vi "Process Message.vi"(8 "error in (no error)":errorcluster, 11 "Message Transport in":refnum<class "Message Transport.lvclass">) -> (0 "error out":errorcluster, 2 "Action":refnum<class "Action.lvclass">, 3 "Message Transport out":refnum<class "Message Transport.lvclass">)   [LabVIEW 2018, in "Message Transport.lvclass"]
uses:
  Message Transport.lvclass
  Action_class/Action.lvclass
  Message Transport.lvclass/Message Transport.ctl
  Message_class/Message.lvclass/Message.ctl
  Communication_class/Get Message Queue.vi
  Message_class/Get Action.vi
  Message_class/Message.lvclass
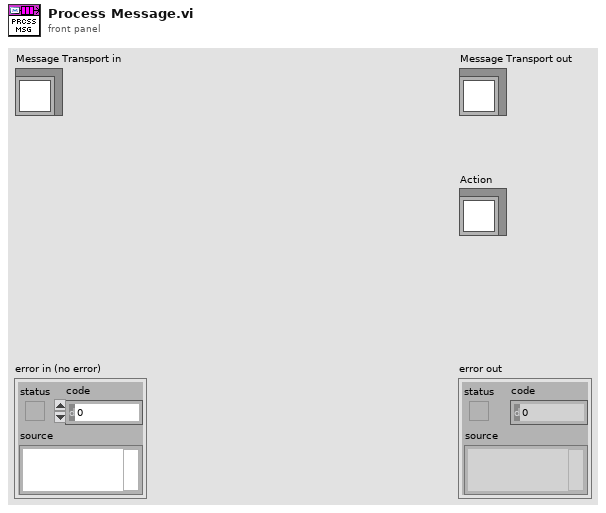
[diagram p1: front panel]
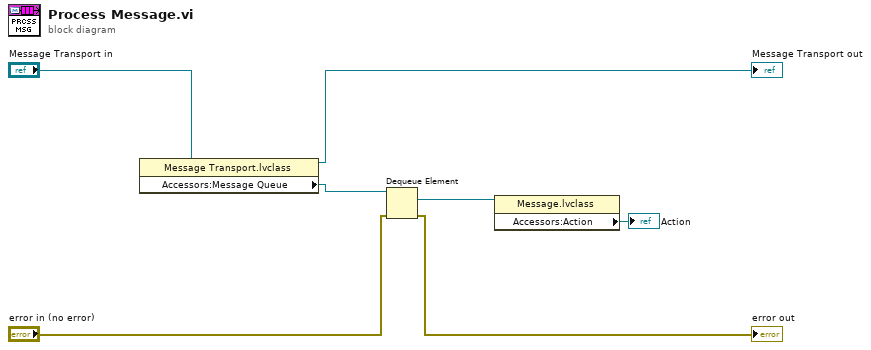
[diagram p0: block diagram]
diagram:
  n1 = property class="Message Transport.lvclass"(reference="Message Transport in") -> (reference out=→"Message Transport out":refnum<class "Message Transport.lvclass">, "Accessors:Message Queue"=w6:refnum<queue>)  [unwired: 1 in, 1 out]
  n2 = Dequeue Element(queue=w6, error in (no error)="error in (no error)") -> (element=w2:refnum<class "Message.lvclass">, error out=→"error out":errorcluster)  [unwired: 1 in, 2 out]
  n3 = property class="Message.lvclass"(reference=w2) -> ("Accessors:Action"=→"Action":refnum<class "Action.lvclass">)  [unwired: 1 in, 2 out]
